vi "使用范例_当前vi截屏.vi"() -> ()   [LabVIEW 2020]
panel:
  in  "存储路径":path=path "D:/"
  in  "文件序号":string
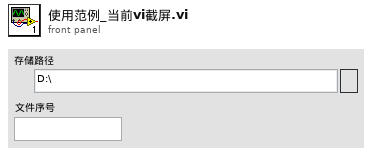
[diagram p1: front panel]
types:
  T1 = typedef "imagedata.ctl" = cluster{"image type":i32, "image depth":i32, "image":u8[], "mask":u8[], "colors":u32[], "Rectangle":cluster{"left":i16, "top":i16, "right":i16, "bottom":i16}}
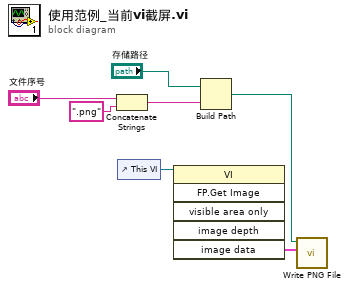
[diagram p0: block diagram]
diagram:
  n1 = Concatenate Strings("文件序号", ".png") -> (w3:string)
  n2 = control-ref of="This VI"() -> (w5:refnum<vi>)
  n3 = invoke class="VI" method="FP.Get Image"(reference=w5) -> ("image data"=w6:T1)  [unwired: 5 in, 5 out]
  n4 = Build Path(base path="存储路径", name or relative path=w3) -> (appended path=w7:path)
  n5 = call <vilib>:"Write PNG File.vi"("image data"=w6, "path to PNG file"=w7) -> ()  [unwired: 8 in, 2 out]
